vi "tcp_stop.vi"(11 "Data":T1) -> ()   [LabVIEW 2018]
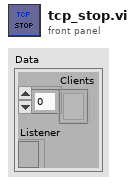
[diagram p1: front panel]
types:
  T1 = cluster{"Clients":refnum<k5>[], "Listener":refnum<k5>}
  T2 = enum16{"Initialize", "Status Check", "Send Data", "Stop"}
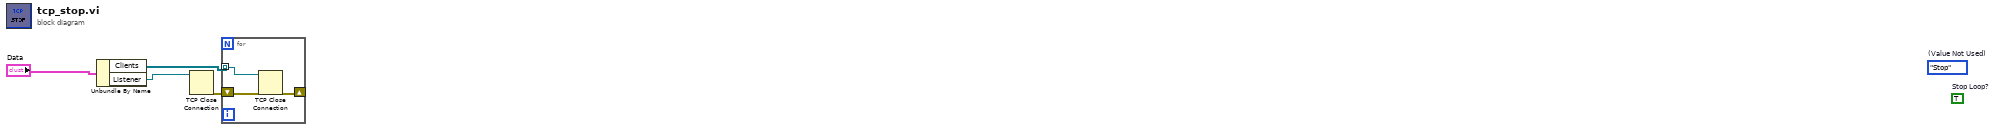
[diagram p0: block diagram]
diagram:
  (unwired) T2."Stop"  # (Value Not Used)
  (unwired) TRUE  # Stop Loop?
  n1 = Unbundle By Name("Data") -> ("Clients"=w4:refnum<k5>[], "Listener"=w2:refnum<k5>)
  n2 = TCP Close Connection(connection ID=w2) -> (error out=w3:errorcluster)  [unwired: 2 in, 1 out]
  n3 = for {
    shift-right: [w6] -> _
    shift-left: w3 -> [w7]
    tunnel: w4 -> [w5] mode=indexing
    n4 = TCP Close Connection(connection ID=w5, error in (no error)=w7) -> (error out=w6:errorcluster)  [unwired: 1 in, 1 out]
  }
